vi "LSCI332 GetManOutput.vi"(0 "VISA Rsrc":refnum<visa-resource-name>="GPIB0::12::INSTR", 5 "Boucle(1)":u32(ring) caption="Boucle" items=["Boucle 1", "Boucle 2"], 11 "error in":errorcluster) -> (4 "ManOutput":dbl caption="Manual Output %" format="%#.2g", 15 "error out":errorcluster)   [LabVIEW 2012]
doc: "Ce Vi nterroge l'instrument sur la valeur de \"Manual output\" de chauffage actuelle, en %."
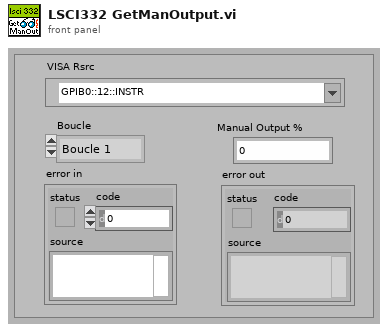
[diagram p1: front panel]
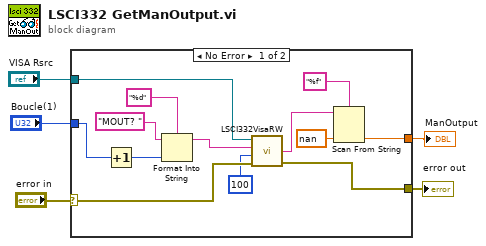
[diagram p0: block diagram]
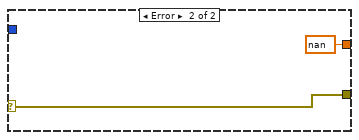
[diagram p2: hidden frame]
diagram:
  n1 = case shown="No Error" "error in" {
    selector: "error in" -> [w17 w20]
    tunnel: [w15 w20] -> w5
    tunnel: "VISA Rsrc" -> [w18 _]
    tunnel: "Boucle(1)" -> [w14 _]
    tunnel: [w10 nan ("default value 1")] -> w1
    frame No Error {
      n2 = Increment(x=w14) -> (x+1=w6:u32)
      n3 = Format Into String(format string="%d", initial string="MOUT? ", w6) -> (resulting string=w12:string)  [unwired: 1 in, 1 out]
      n4 = call <userlib>:"LSCI332VisaRW.vi"("error in (no error)"=w17, "Nbcaract"=u32 100, "ChaineCom"=w12, "VISA Rsrc"=w18) -> ("error out"=w15:errorcluster, "ChaineRep"=w11:string)  [unwired: 3 in, 2 out]
      n5 = Scan From String(format string="%f", input string=w11, default 1=nan ("default value 1")) -> (output 1=w10:dbl)  [unwired: 2 in, 3 out]
    }
    frame Error {
    }
  }
  "error out" <- w5
  "ManOutput" <- w1
